vi "Soft Stops Rate.vi"(0 "Motor In":dbl=0.04, 1 "Disable Softstops":bool, 2 "Disable Motor":bool, 3 "correlation":bool=TRUE, 5 "Sense":dbl, 9 "Target":dbl=-10.0, 12 "Lo Rate":dbl=0.02, 13 "Margin":dbl=1.0, 14 "Motor Coerce":dbl=1.0) -> (4 "Motor Out":dbl, 10 "At Lo":bool, 15 "At Hi":bool)   [LabVIEW 2012]
panel:
  in  "Set Point":dbl=-10.0
  in  "Margin 2":dbl=1.0
  in  "Rate Sense":dbl
  in  "Lo Rate":dbl=400.0
  in  "gain 2":dbl(knob)=0.0010163019655977424 scale=0.0..0.1
  out "val 2":dbl
  in  "dir 2":bool
  in  "zero 2":bool
  in  "Position Sense":dbl
  in  "zero":bool
  in  "dir":bool
  out "val":dbl
  in  "gain":dbl(knob)=0.0010163019655977424 scale=0.0..0.1
  in  "Rate":dbl=400.0
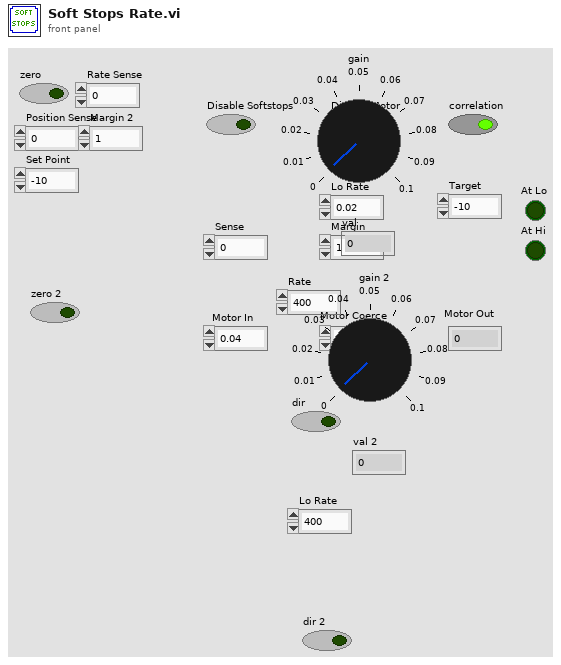
[diagram p1: front panel]
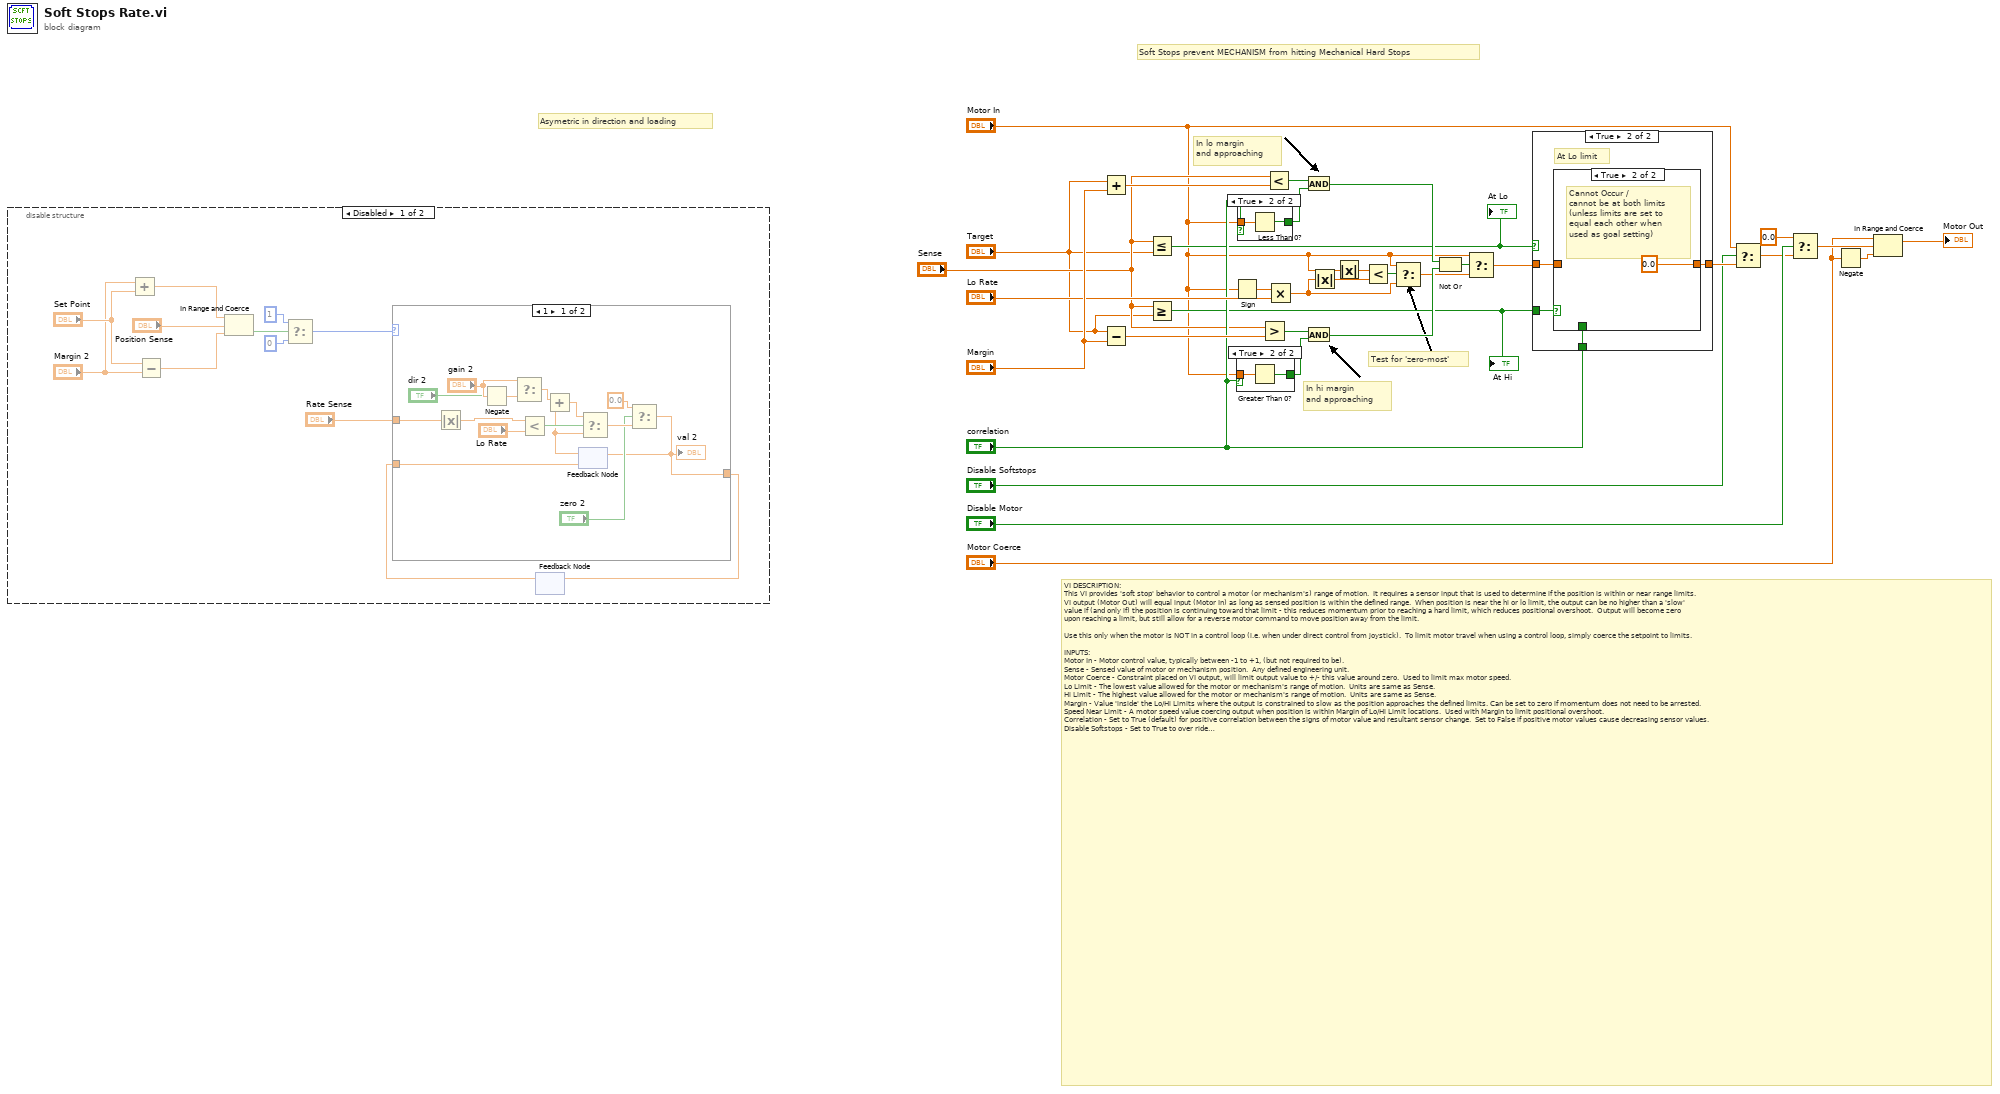
[diagram p0: block diagram]
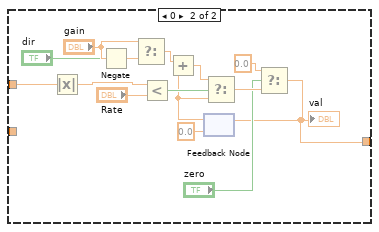
[diagram p2: hidden frame]
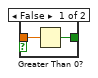
[diagram p4: hidden frame]
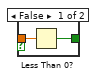
[diagram p5: hidden frame]
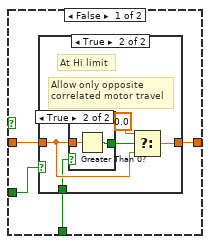
[diagram p6: hidden frame]
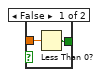
[diagram p8: hidden frame]
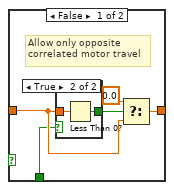
[diagram p9: hidden frame]
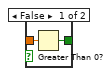
[diagram p10: hidden frame]
diagram:
  # "Asymetric in direction and loading"
  # "In hi margin\nand approaching"
  # "In lo margin\nand approaching"
  # "Test for 'zero-most'"
  # "VI DESCRIPTION:\nThis VI provides 'soft stop' behavior to control a motor (or mechanism's) range of motion.  It requires a sensor input that is used to determine if the position is within or near range limits.\nVI output (Motor Out) will equal input (Motor In) as long as sensed position is within the defined range.  When position is near the hi or lo limit, the output can be no higher than a 'slow'\nvalue if (and only if) the position is continuing toward that limit - this reduces momentum prior to reaching a hard limit, which reduces positional overshoot.  Output will become zero \nupon reaching a limit, but still allow for a reverse motor command to move position away from the limit.\n\nUse this only when the motor is NOT in a control loop (i.e. when under direct control from joystick).  To limit motor travel when using a control loop, simply coerce the setpoint to limits.\n\nINPUTS:\nMotor In - Motor control value, typically between -1 to +1, (but not required to be).\nSense - Sensed value of motor or mechanism position.  Any defined engineering unit.\nMotor Coerce - Constraint placed on VI output, will limit output value to +/- this value around zero.  Used to limit max motor speed.\nLo Limit - The lowest value allowed for the motor or mechanism's range of motion.  Units are same as Sense.\nHi Limit - The highest value allowed for the motor or mechanism's range of motion.  Units are same as Sense.\nMargin - Value 'inside' the Lo/Hi Limits where the output is constrained to slow as the position approaches the defined limits. Can be set to zero if momentum does not need to be arrested.\nSpeed Near Limit - A motor speed value coercing output when position is within Margin of Lo/Hi Limit locations.  Used with Margin to limit positional overshoot.\nCorrelation - Set to True (default) for positive correlation between the signs of motor value and resultant sensor change.  Set to False if positive motor values cause decreasing sensor values.\nDisable Softstops - Set to True to over ride the softstop behavor and pass Motor In directly to Motor Out.\nDisable Motor - Set to True to send value zero to Motor Output.  If both Disables are selected, Disable Motor takes precedence over Disable Softstops.\n\nOUTPUTS:\nMotor Out - Motor control value modified by VI behavior.\nAt Lo - Boolean indicating status of sensed position, True if equal or lower than Lo Limit.\nAt Hi - Boolean indicating status of sensed position, True if equal or higher than Hi Limit.\n\nIMPLEMENTATION:\nDo not use in a control loop, instead use setpoint coercion for this situation.  For direct motor control:\nDetermine the correlation of the mechanical arrangement; if positive motor values cause increasing sensor values, set Correlation to True.\nDetermine the physical limits of the mechanism and set Lo and Hi Limits just short of these limits, by an amount that will accomodate any small overshoot that might remain after tuning.\nTo limit positional overshoot, create a region just inside each limit to slow the motor by setting Margin.\nSet Speed Near Limit to a value slow enough to bring the mechanism to a stop prior to reaching physical limits.\nSet Motor Coerce to the maximum speed that the mechanism is allowed to travel.\nExperimentally determine values that minimize the Margin region and maximize Speed Near Limit, without striking the mechanism's physical limits when approaching at full speed.\n\n\nFIRST Team 836, RoboBees"
  # "Soft Stops prevent MECHANISM from hitting Mechanical Hard Stops"
  n1 = disable-structure shown="Disabled" {
    frame Disabled {
      n2 = Add(x="Margin 2", y="Set Point") -> (x+y=w39:dbl)
      n3 = Subtract(x="Set Point", y="Margin 2") -> (x-y=w42:dbl)
      n4 = In Range and Coerce(upper limit=w39, x="Position Sense", lower limit=w42) -> (In Range?=w37:bool)  [unwired: 1 out]
      n5 = Select(t=1, s=w37, f=0) -> (s? t:f=w34:i32)
      n6 = feedback #1() -> (w43:dbl)  [unwired: 1 in]
      n7 = case shown="1" w34 {
        tunnel: "Rate Sense" -> [w46 w62]
        tunnel: [w47 w61] -> w44
        tunnel: w43 -> [w48 _]
        frame 1 {
          n8 = Absolute Value(x=w46) -> (abs(x)=w56:dbl)
          n9 = Negate(x="gain 2") -> (-x=w52:dbl)
          n10 = Select(t="gain 2", s="dir 2", f=w52) -> (s? t:f=w53:dbl)
          n11 = Less?(x=w56, y="Lo Rate") -> (x < y?=w59:bool)
          n12 = feedback #2(w48) -> (w57:dbl)
          n13 = Add(x=w53, y=w57) -> (x+y=w58:dbl)
          n14 = Select(t=w58, s=w59, f=w57) -> (s? t:f=w55:dbl)
          n15 = Select(t=0.0, s="zero 2", f=w55) -> (s? t:f=w47:dbl)
          "val 2" <- w47
          n16 = feedback-in #2(w47) -> ()
        }
        frame 0 {
          n17 = Absolute Value(x=w62) -> (abs(x)=w70:dbl)
          n18 = Negate(x="gain") -> (-x=w66:dbl)
          n19 = Select(t="gain", s="dir", f=w66) -> (s? t:f=w67:dbl)
          n20 = Less?(x=w70, y="Rate") -> (x < y?=w73:bool)
          n21 = feedback #3(0.0) -> (w71:dbl)
          n22 = Add(x=w67, y=w71) -> (x+y=w72:dbl)
          n23 = Select(t=w72, s=w73, f=w71) -> (s? t:f=w69:dbl)
          n24 = Select(t=0.0, s="zero", f=w69) -> (s? t:f=w61:dbl)
          "val" <- w61
          n25 = feedback-in #3(w61) -> ()
        }
      }
      n26 = feedback-in #1(w44) -> ()
    }
    frame Enabled {
    }
  }
  n27 = Add(x="Target", y="Margin") -> (x+y=w19:dbl)
  n28 = Subtract(x="Target", y="Margin") -> (x-y=w16:dbl)
  n29 = Less Or Equal?(x="Sense", y="Target") -> (x <= y?=w5:bool)
  "At Lo" <- w5
  n30 = Greater Or Equal?(x="Sense", y="Target") -> (x >= y?=w4:bool)
  "At Hi" <- w4
  n31 = Sign(1:"Motor In") -> (0:w23:dbl)
  n32 = case shown="True" "correlation" {
    tunnel: [w76 w78] -> w15
    tunnel: "Motor In" -> [w77 w79]
    frame False {
      n33 = Less Than 0?(x=w77) -> (x < 0?=w76:bool)
    }
    frame True {
      n34 = Greater Than 0?(x=w79) -> (x > 0?=w78:bool)
    }
  }
  n35 = case shown="True" "correlation" {
    tunnel: [w81 w83] -> w18
    tunnel: "Motor In" -> [w80 w82]
    frame False {
      n36 = Greater Than 0?(x=w80) -> (x > 0?=w81:bool)
    }
    frame True {
      n37 = Less Than 0?(x=w82) -> (x < 0?=w83:bool)
    }
  }
  n38 = Greater?(x="Sense", y=w16) -> (0:w17:bool)
  n39 = Less?(x="Sense", y=w19) -> (x < y?=w20:bool)
  n40 = Multiply(x=w23, y="Lo Rate") -> (x*y=w6:dbl)
  n41 = And(x=w20, y=w18) -> (x .and. y?=w14:bool)
  n42 = And(x=w17, y=w15) -> (x .and. y?=w13:bool)
  n43 = Absolute Value(x=w6) -> (abs(x)=w8:dbl)
  n44 = Absolute Value(x="Motor In") -> (abs(x)=w9:dbl)
  n45 = Less?(x=w9, y=w8) -> (x < y?=w10:bool)
  n46 = Select(t="Motor In", s=w10, f=w6) -> (s? t:f=w7:dbl)
  n47 = Not Or(1:w13, 2:w14) -> (0:w12:bool)
  n48 = Select(t="Motor In", s=w12, f=w7) -> (s? t:f=w21:dbl)
  n49 = case shown="True" w5 {
    tunnel: [w86 w100] -> w32
    tunnel: w21 -> [w87 w101]
    tunnel: "correlation" -> [w85 w99]
    tunnel: w4 -> [w84 w98]
    frame False {
      n50 = case shown="True" w84 {
        tunnel: w87 -> [w88 w91]
        tunnel: [w88 w90] -> w86
        tunnel: w85 -> [_ w89]
        frame False {
          # "At neither limit"
        }
        frame True {
          # "Allow only opposite\ncorrelated motor travel"
          # "At Hi limit"
          n51 = case shown="True" w89 {
            tunnel: [w95 w96] -> w93
            tunnel: w91 -> [w94 w97]
            frame False {
              n52 = Less Than 0?(x=w94) -> (x < 0?=w95:bool)
            }
            frame True {
              n53 = Greater Than 0?(x=w97) -> (x > 0?=w96:bool)
            }
          }
          n54 = Select(t=0.0, s=w93, f=w91) -> (s? t:f=w90:dbl)
        }
      }
    }
    frame True {
      # "At Lo limit"
      n55 = case shown="True" w98 {
        tunnel: w101 -> [w103 _]
        tunnel: [w104 0.0 ("Turret Yaw Control")] -> w100
        tunnel: w99 -> [w102 _]
        frame False {
          # "Allow only opposite\ncorrelated motor travel"
          n56 = case shown="True" w102 {
            tunnel: [w108 w109] -> w106
            tunnel: w103 -> [w107 w110]
            frame False {
              n57 = Greater Than 0?(x=w107) -> (x > 0?=w108:bool)
            }
            frame True {
              n58 = Less Than 0?(x=w110) -> (x < 0?=w109:bool)
            }
          }
          n59 = Select(t=0.0, s=w106, f=w103) -> (s? t:f=w104:dbl)
        }
        frame True {
          # "Cannot Occur / \ncannot be at both limits\n(unless limits are set to\nequal each other when\nused as goal setting)"
        }
      }
    }
  }
  n60 = Select(t="Motor In", s="Disable Softstops", f=w32) -> (s? t:f=w25:dbl)
  n61 = Select(t=0.0, s="Disable Motor", f=w25) -> (s? t:f=w31:dbl)
  n62 = Negate(x="Motor Coerce") -> (-x=w30:dbl)
  n63 = In Range and Coerce(upper limit="Motor Coerce", x=w31, lower limit=w30) -> (coerced(x)=→"Motor Out":dbl)  [unwired: 1 out]
